vi "RB2 parse the data.vi"(0 "Nav String":string="$,G,154,395,B,181,365,R,150,368,N,185,392,V,311,47,W,35,87,X,195,214,Y,517,324,Z,43,325,S,14,3,553\r", 1 "Jeep":string="G") -> (2 "Jeep Data":cluster{"Header":string, i32, i32}, 3 "Time":cluster{i32, i32, i32}, 4 "Post String":string, 5 "Valid?":bool)   [LabVIEW 2012]
doc: "This VI find the position of the tug, X, Y and Heading convered into grid values. The position values are positions on the occupancy grid, the heading is in degrees. It also finds the buoy locations in grid values and the time in hrs, min , secs."
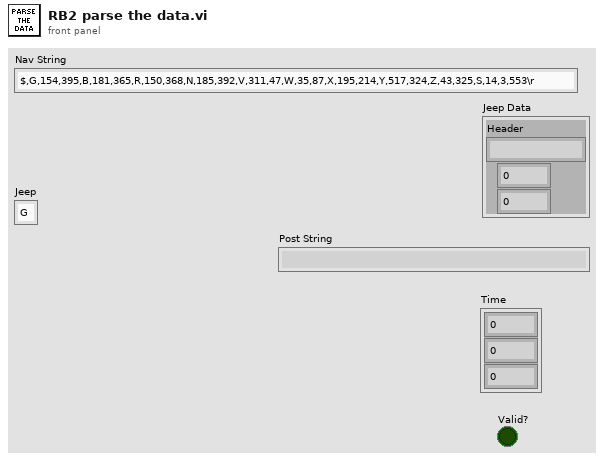
[diagram p1: front panel]
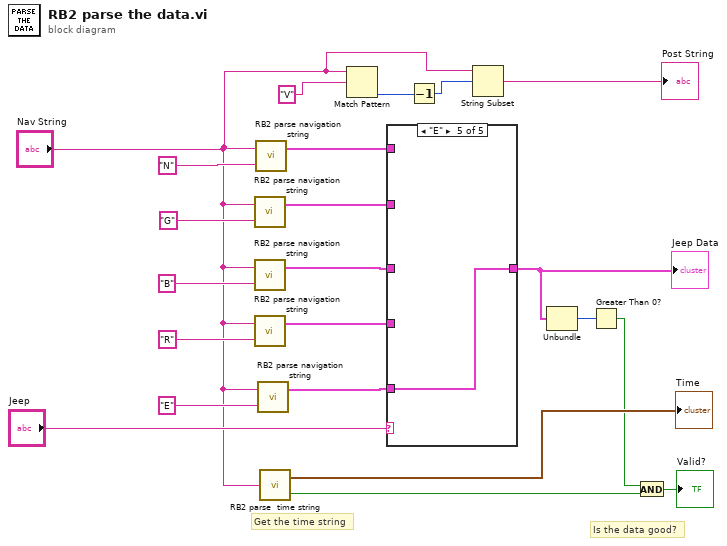
[diagram p0: block diagram]
diagram:
  # "Is the data good?"
  # "Get the time string"
  n1 = call "RB2 parse navigation string.vi"("Header"="G", "Nav String"="Nav String") -> ("Jeep Data"=w15:cluster{"Header":string, i32, i32})  [unwired: 1 out]
  n2 = call "RB2 parse navigation string.vi"("Header"="B", "Nav String"="Nav String") -> ("Jeep Data"=w13:cluster{"Header":string, i32, i32})  [unwired: 1 out]
  n3 = call "RB2 parse navigation string.vi"("Header"="R", "Nav String"="Nav String") -> ("Jeep Data"=w12:cluster{"Header":string, i32, i32})  [unwired: 1 out]
  n4 = call "RB2 parse navigation string.vi"("Header"="N", "Nav String"="Nav String") -> ("Jeep Data"=w16:cluster{"Header":string, i32, i32})  [unwired: 1 out]
  n5 = call "RB2 parse navigation string.vi"("Header"="E", "Nav String"="Nav String") -> ("Jeep Data"=w11:cluster{"Header":string, i32, i32})  [unwired: 1 out]
  n6 = call "RB2 parse  time string.vi"("Nav String"="Nav String") -> ("output cluster"=→"Time":cluster{i32, i32, i32}, "Valid?"=w7:bool)
  n7 = Match Pattern(string="Nav String", regular expression="V") -> (offset past match=w4:i32)  [unwired: 1 in, 3 out]
  n8 = case shown="\"E\"" "Jeep" {
    tunnel: w16 -> [w23 _ _ _ _]
    tunnel: w15 -> [_ w24 _ _ _]
    tunnel: w13 -> [_ _ w25 _ _]
    tunnel: w12 -> [_ _ _ w26 _]
    tunnel: w11 -> [_ _ _ _ w27]
    tunnel: [w23 w24 w25 w26 w27] -> w10
    frame "N", Default {
    }
    frame "G" {
    }
    frame "B" {
    }
    frame "R" {
    }
    frame "E" {
    }
  }
  "Jeep Data" <- w10
  n9 = Decrement(x=w4) -> (x-1=w3:i32)
  n10 = String Subset(string="Nav String", offset (0)=w3) -> (substring=→"Post String":string)  [unwired: 1 in]
  n11 = Unbundle(w10) -> (w9:i32)  [unwired: 2 out]
  n12 = Greater Than 0?(x=w9) -> (x > 0?=w6:bool)
  n13 = And(x=w6, y=w7) -> (x .and. y?=→"Valid?":bool)
